vi "Reto(for).vi"() -> ()   [LabVIEW 2020]
panel:
  in  "Parar":bool
  in  "milliseconds to wait":u32
  in  "Numeric":i32
  out "Random":dbl
  out "Iteraciones":i32
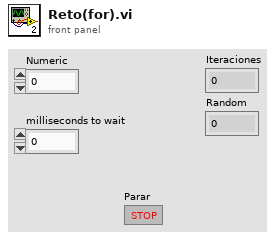
[diagram p1: front panel]
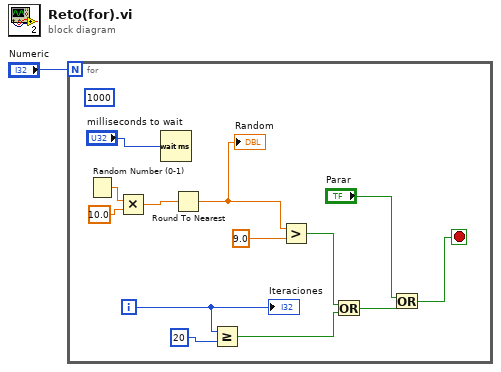
[diagram p0: block diagram]
diagram:
  n1 = for {
    N: "Numeric" -> [_]
    i -> [w11]
    stop <- w4 stop-if-true
    (unwired) u32 1000 ("milliseconds to wait")
    n2 = Random Number (0-1)() -> (number: 0 to 1=w14:dbl)
    n3 = Multiply(x=w14, y=10.0) -> (x*y=w12:dbl)
    n4 = Wait (ms)(milliseconds to wait="milliseconds to wait") -> ()  [unwired: 1 out]
    n5 = Round To Nearest(number=w12) -> (nearest integer value=w3:dbl)
    "Random" <- w3
    n6 = Greater Or Equal?(x=w11, y=20) -> (x >= y?=w9:bool)
    n7 = Greater?(x=w3, y=9.0 ("x")) -> (0:w8:bool)
    n8 = Or(x=w8, y=w9) -> (x .or. y?=w6:bool)
    n9 = Or(x="Parar", y=w6) -> (x .or. y?=w4:bool)
    "Iteraciones" <- w11
  }
